vi "Create.vi"(6 "Category":i32, 7 "ID":i32, 8 "Balance":dbl, 9 "Amount":dbl, 10 "Description":string, 11 "Date":timestamp) -> (3 "Banking Record":refnum<class "Banking Record.lvclass">)   [LabVIEW 2018, in "Banking Record.lvclass"]
uses:
  Banking Record.lvclass
  Banking Record.lvclass/Banking Record.ctl
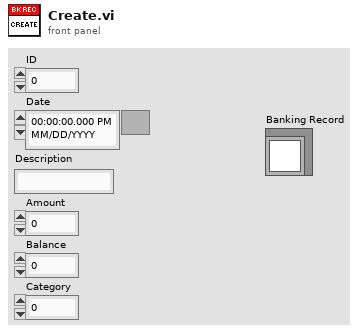
[diagram p1: front panel]
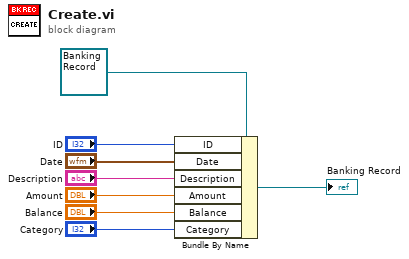
[diagram p0: block diagram]
diagram:
  n1 = Bundle By Name(cluster=refnum<class "Banking Record.lvclass"> refnum ("Banking Record.lvclass"), "ID"="ID", "Date"="Date", "Description"="Description", "Amount"="Amount", "Balance"="Balance", "Category"="Category") -> (→"Banking Record":refnum<class "Banking Record.lvclass">)
